vi "Configure Channels.vi"(8 "error in":errorcluster, 11 "Thermometer DAQmx RTD Cont CFG in":refnum<class "Thermometer DAQmx RTD Cont CFG.lvclass">) -> (0 "error out":errorcluster, 3 "Thermometer DAQmx RTD Cont CFG out":refnum<class "Thermometer DAQmx RTD Cont CFG.lvclass">)   [LabVIEW 2023, in "Thermometer DAQmx RTD Cont CFG.lvclass"]
uses:
  Thermometer DAQmx RTD Cont CFG.lvclass
  D:/git/HAL/HAL GOOP4/Configuration/Configuration JSON/Configuration JSON Base/CFG JSON.lvclass
  D:/git/HAL/HAL GOOP4/DAQmx/DAQmx Base CFG/DAQmx Base CFG.lvclass
  DAQmx/DAQmx Base CFG/DAQmx Base CFG.lvclass/DAQmx Base CFG.ctl
  Configuration/Configuration JSON/Configuration JSON Base/CFG JSON.lvclass/CFG JSON.ctl
  Thermometer DAQmx RTD Cont CFG.lvclass/Thermometer DAQmx RTD Cont CFG.ctl
  062e36a0-2821-4acd-afc3-503ce041c10d.vi
  <vilib>/JDP Science/JSONtext/Find Item.vi
  <vilib>/JDP Science/JSONtext/Next JSON Value.vi
  <vilib>/JDP Science/JSONtext/String Subset.vi
  <vilib>/JDP Science/JSONtext/Parsing/Advance past next JSON Value (inlined COPY).vi
  <vilib>/JDP Science/JSONtext/Parsing/Advance past whitespace.vi
  <vilib>/JDP Science/JSONtext/Parsing/Advance past String.vi
  <vilib>/JDP Science/JSONtext/Parsing/Advance past Number.vi
  <vilib>/JDP Science/JSONtext/Parsing/Advance past Line Ending.vi
  <vilib>/JDP Science/JSONtext/Parsing/Parse Full Path or Item Name.vi
  <vilib>/JDP Science/JSONtext/Parsing/Advance past Array.vi
  <vilib>/JDP Science/JSONtext/Parsing/Advance past Object.vi
  <vilib>/JDP Science/JSONtext/support/Error Cluster From Code.vi
  <vilib>/JDP Science/JSONtext/Offset/Find Item Locations by Path.vi
  <vilib>/JDP Science/JSONtext/JSON text to Variant.vi
  <vilib>/DAQmx/create/channels.llb/DAQmx Create Channel (AI-Temperature-RTD).vi
  <vilib>/JDP Science/JSONtext/LVClass Serializer/JSONtext LVClass Serializer.lvclass
  Configuration/Configuration JSON/Configuration JSON Base/CFG JSON.lvclass
  DAQmx/DAQmx Base CFG/DAQmx Base CFG.lvclass
panel:
  out "units":i32(ring)=10143 items=["Deg C"=10143, "Deg F"=10144, "Kelvins"=10325, "Deg R"=10145, "From Custom Scale"=10065]
  out "rtd type":i32(ring)=12481 items=["Pt3750"=12481, "Pt3851"=10071, "Pt3911"=12482, "Pt3916"=10069, "Pt3920"=10053, "Pt3928"=12483, "Custom"=10137]
  out "current excitation source":i32(ring)=10167 items=["Internal"=10200, "External"=10167, "None"=10230]
  out "resistance cfg":i32(ring)=4 items=["2-Wire"=2, "3-Wire"=3, "4-Wire"=4]
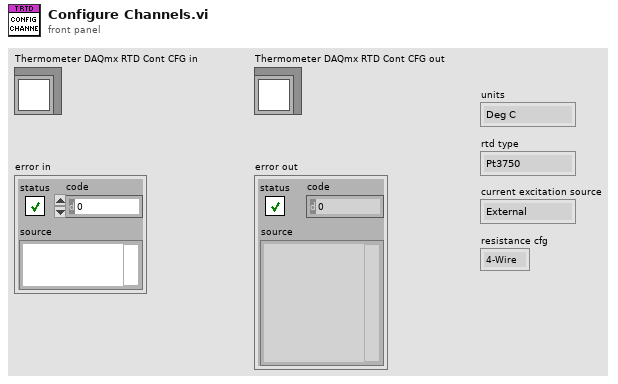
[diagram p1: front panel]
types:
  T1 = cluster{"Name":string, "Enabled":bool, "Minimum Value":dbl, "Maximum Value":dbl, "Resistance CFG":string, "R0":dbl, "Excitation Current":dbl, "Units":string, "Excitation Current Src":string, "RTD Type":string}[]
  T2 = typedef "LVStringsAndValuesArrayTypeDef_I32.ctl" = cluster{"String":string, "Value":i32}[]
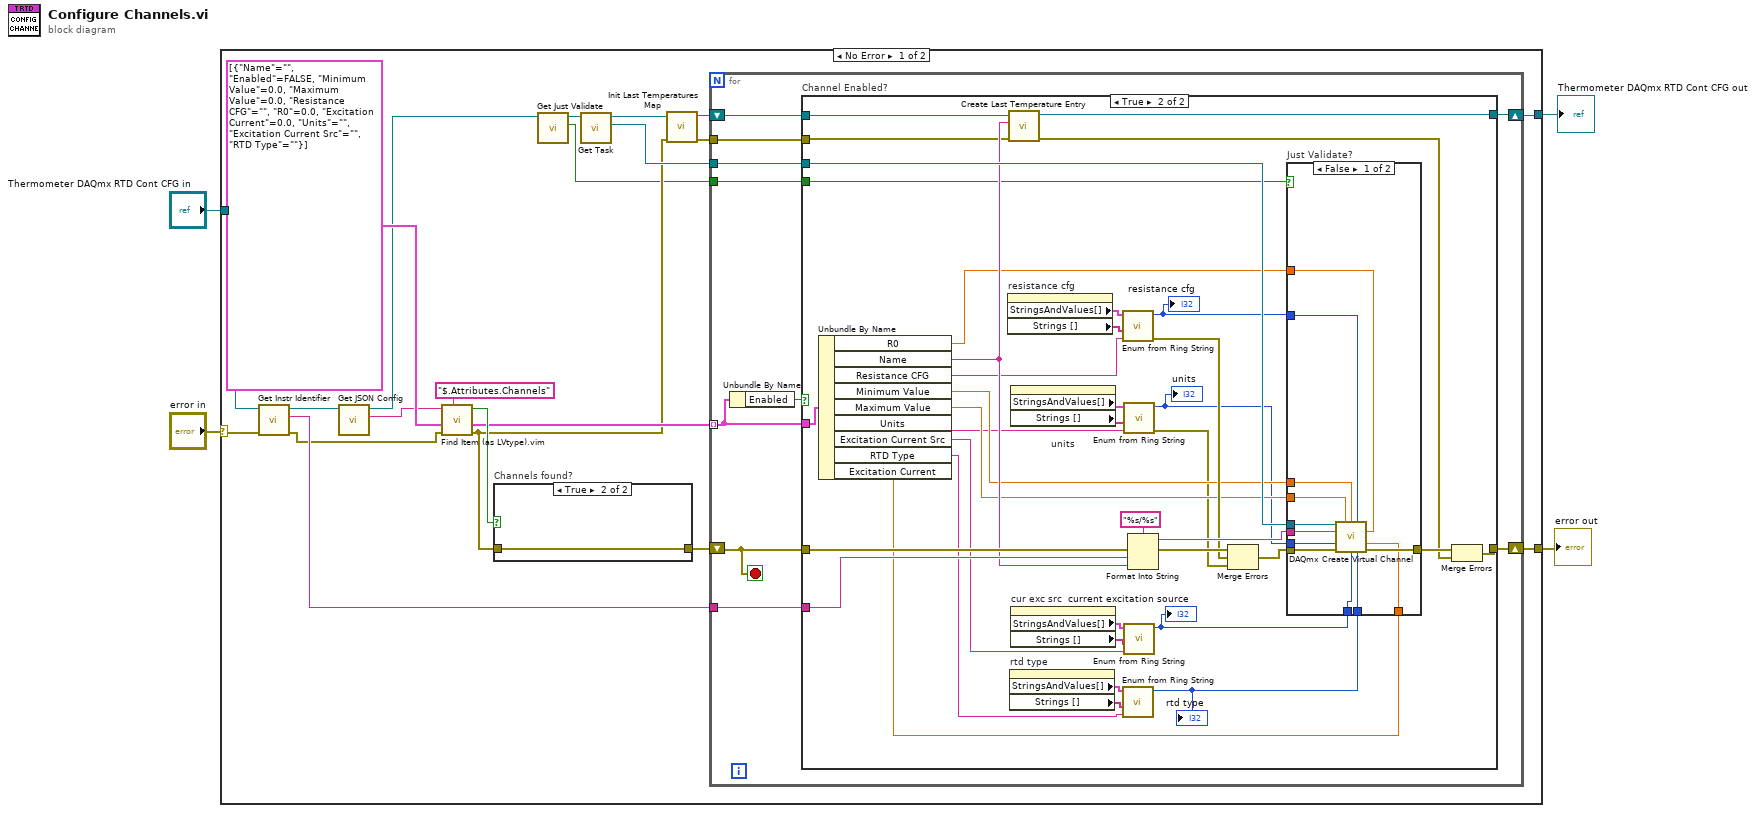
[diagram p0: block diagram]
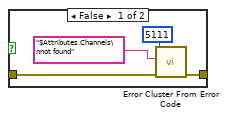
[diagram p2: hidden frame]
diagram:
  n1 = case shown="No Error" "error in" {
    selector: "error in" -> [w19 w94]
    tunnel: "Thermometer DAQmx RTD Cont CFG in" -> [w15 w95]
    tunnel: [w20 w94] -> w1
    tunnel: [w14 w95] -> w2
    frame No Error {
      n2 = call-dynamic "Get Instr Identifier.vi"("error in (no error)"=w19, "Configuration Base in"=w15) -> ("error out"=w5:errorcluster, "Instr Ident"=w21:string, "Configuration Base out"=w22:refnum<class "Thermometer DAQmx RTD Cont CFG.lvclass">)  [unwired: 7 in]
      n3 = call "Get JSON Config.vi"("CFG Base in"=w22) -> ("<JSON>Config>"=w18:string, "CFG Base out"=w9:refnum<class "Thermometer DAQmx RTD Cont CFG.lvclass">)  [unwired: 9 in]
      n4 = call "Find Item (as LVtype).vim"("$Path or Item Name"="$.Attributes.Channels", "error in (no error)"=w5, "Data Type and Default Value"=T1 [{"Name"="", "Enabled"=FALSE, "Minimum Value"=0.0, "Maximum Value"=0.0, "Resistance CFG"="", "R0"=0.0, "Excitation Current"=0.0, "Units"="", "Excitation Current Src"="", "RTD Type"=""}], "JSON"=w18) -> ("error out"=w12:errorcluster, "Data"=w16:T1, "Found"=w24:bool)  [unwired: 4 in, 1 out]
      n5 = case "Channels found?" shown="True" w24 {
        tunnel: w12 -> [w26 w30]
        tunnel: [w27 w30] -> w13
        frame False {
          n6 = call <vilib>:"Error Cluster From Error Code.vi"("error in (no error)"=w26, "error message (\"\")"="$Attributes.Channels\nnot found" ("error message (\"\")"), "error code (0)"=5111) -> ("error out"=w27:errorcluster)  [unwired: 6 in]
        }
        frame True {
        }
      }
      n7 = call "Get Just Validate.vi"("CFG JSON Base in"=w9) -> ("Just Validate"=w10:bool, "CFG JSON Base out"=w8:refnum<class "Thermometer DAQmx RTD Cont CFG.lvclass">)  [unwired: 9 in]
      n8 = call "Get Task.vi"("DAQmx Base CFG in"=w8) -> ("Task"=w17:refnum<k21>, "DAQmx Base CFG out"=w7:refnum<class "Thermometer DAQmx RTD Cont CFG.lvclass">)  [unwired: 9 in]
      n9 = call "Init Last Temperatures Map.vi"("error in"=w12, "Thermometer DAQmx RTD Cont CFG in"=w7) -> ("error out"=w11:errorcluster, "Thermometer DAQmx RTD Cont CFG out"=w6:refnum<class "Thermometer DAQmx RTD Cont CFG.lvclass">)  [unwired: 8 in]
      n10 = for {
        tunnel: w16 -> [w37] mode=indexing
        shift-right: [w40] -> w20
        shift-left: w13 -> [w39]
        tunnel: w21 -> [w38]
        tunnel: w17 -> [w36]
        shift-right: [w35] -> w14
        shift-left: w6 -> [w34]
        tunnel: w11 -> [w32]
        tunnel: w10 -> [w31]
        stop <- w39 stop-if-true
        n11 = Unbundle By Name(w37) -> ("Enabled"=w33:bool)
        n12 = case "Channel Enabled?" shown="True" w33 {
          tunnel: [w42 w78] -> w40
          tunnel: w39 -> [w42 w75]
          tunnel: w38 -> [_ w74]
          tunnel: w37 -> [_ w80]
          tunnel: [w41 w70] -> w35
          tunnel: w36 -> [_ w77]
          tunnel: w34 -> [w41 w60]
          tunnel: w32 -> [_ w62]
          tunnel: w31 -> [_ w61]
          frame False {
          }
          frame True {
            n13 = Unbundle By Name(w80) -> ("R0"=w59:dbl, "Name"=w69:string, "Resistance CFG"=w68:string, "Minimum Value"=w58:dbl, "Maximum Value"=w57:dbl, "Units"=w54:string, "Excitation Current Src"=w49:string, "RTD Type"=w46:string, "Excitation Current"=w43:dbl)
            n14 = property on="resistance cfg" class="Ring (strict)"() -> ("StringsAndValues[]"=w67:T2, "Strings []"=w66:string[])  [unwired: 2 in, 2 out]
            n15 = call "Create Last Temperature Entry.vi"("error in"=w62, "Channel"=w69, "Thermometer DAQmx RTD Cont CFG in"=w60) -> ("error out"=w71:errorcluster, "Thermometer DAQmx RTD Cont CFG out"=w70:refnum<class "Thermometer DAQmx RTD Cont CFG.lvclass">)  [unwired: 7 in]
            n16 = property on="rtd type" class="Ring (strict)"() -> ("StringsAndValues[]"=w48:T2, "Strings []"=w47:string[])  [unwired: 2 in, 2 out]
            n17 = property on="units" class="Ring (strict)"() -> ("StringsAndValues[]"=w55:T2, "Strings []"=w56:string[])  [unwired: 2 in, 2 out]
            n18 = property on="cur exc src" class="Ring (strict)"() -> ("StringsAndValues[]"=w51:T2, "Strings []"=w50:string[])  [unwired: 2 in, 2 out]
            n19 = call "Enum from Ring String.vi"("String to Match"=w68, "Ring Strings []"=w66, "Ring StringsAndValues[]"=w67) -> ("error out"=w64:errorcluster, "Enum Value"=w63:i32)  [unwired: 7 in]
            "resistance cfg" <- w63
            n20 = call "Enum from Ring String.vi"("String to Match"=w46, "Ring Strings []"=w47, "Ring StringsAndValues[]"=w48) -> ("Enum Value"=w45:i32)  [unwired: 7 in, 1 out]
            "rtd type" <- w45
            n21 = call "Enum from Ring String.vi"("String to Match"=w54, "Ring Strings []"=w56, "Ring StringsAndValues[]"=w55) -> ("error out"=w53:errorcluster, "Enum Value"=w52:i32)  [unwired: 7 in]
            "units" <- w52
            n22 = call "Enum from Ring String.vi"("String to Match"=w49, "Ring Strings []"=w50, "Ring StringsAndValues[]"=w51) -> ("Enum Value"=w44:i32)  [unwired: 7 in, 1 out]
            "current excitation source" <- w44
            n23 = Format Into String(format string="%s/%s", error in=w75, w74, w69) -> (resulting string=w72:string, error out=w73:errorcluster)  [unwired: 1 in]
            n24 = Merge Errors(w73, w64, w53) -> (w65:errorcluster)
            n25 = case "Just Validate?" shown="False" w61 {
              tunnel: w65 -> [w92 w93]
              tunnel: w72 -> [w89 _]
              tunnel: w77 -> [w91 _]
              tunnel: [w90 w93] -> w79
              tunnel: w63 -> [w88 _]
              tunnel: w59 -> [w87 _]
              tunnel: w58 -> [w86 _]
              tunnel: w57 -> [w85 _]
              tunnel: w52 -> [w84 _]
              tunnel: w45 -> [w83 _]
              tunnel: w44 -> [w82 _]
              tunnel: w43 -> [w81 _]
              frame False {
                n26 = call-poly <vilib>:"DAQmx Create Virtual Channel.vi"("task in"=w91, "maximum value"=w85, "minimum value"=w86, "resistance configuration"=w88, "physical channels"=w89, "r0"=w87, "units"=w84, "current excitation value"=w81, "error in"=w92, "current excitation source"=w82, "rtd type"=w83) -> ("error out"=w90:errorcluster)  [unwired: 3 in, 1 out]
              }
              frame True {
              }
            }
            n27 = Merge Errors(w79, w71) -> (w78:errorcluster)
          }
        }
      }
    }
    frame Error {
    }
  }
  "error out" <- w1
  "Thermometer DAQmx RTD Cont CFG out" <- w2
